vi "Format JSON Object.vi"(7 "Alphabetical Sort":bool, 8 "error in (no error)":errorcluster, 9 "Pretty Print?":bool, 10 "JSON elements":string[](array[string]), 11 "Names":string[](array[string])) -> (0 "error out":errorcluster, 3 "JSON Object Text out":string)   [LabVIEW 2017, in "JSONtext.lvlib"]
uses:
  JSONtext.lvlib
  <vilib>/JDP Science/JDP Science Common Utilities/Trim Whitespace__JDP.vi
  quote and escape json string 2.vi
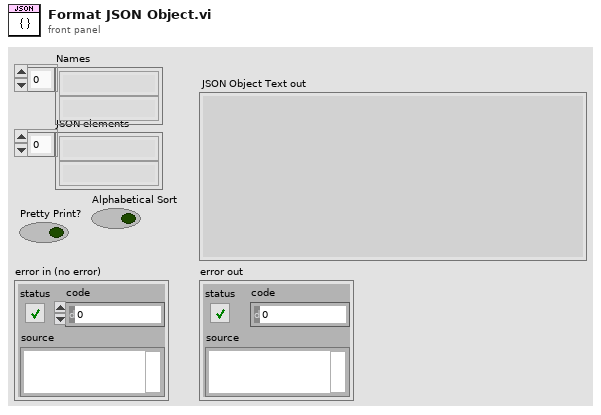
[diagram p1: front panel]
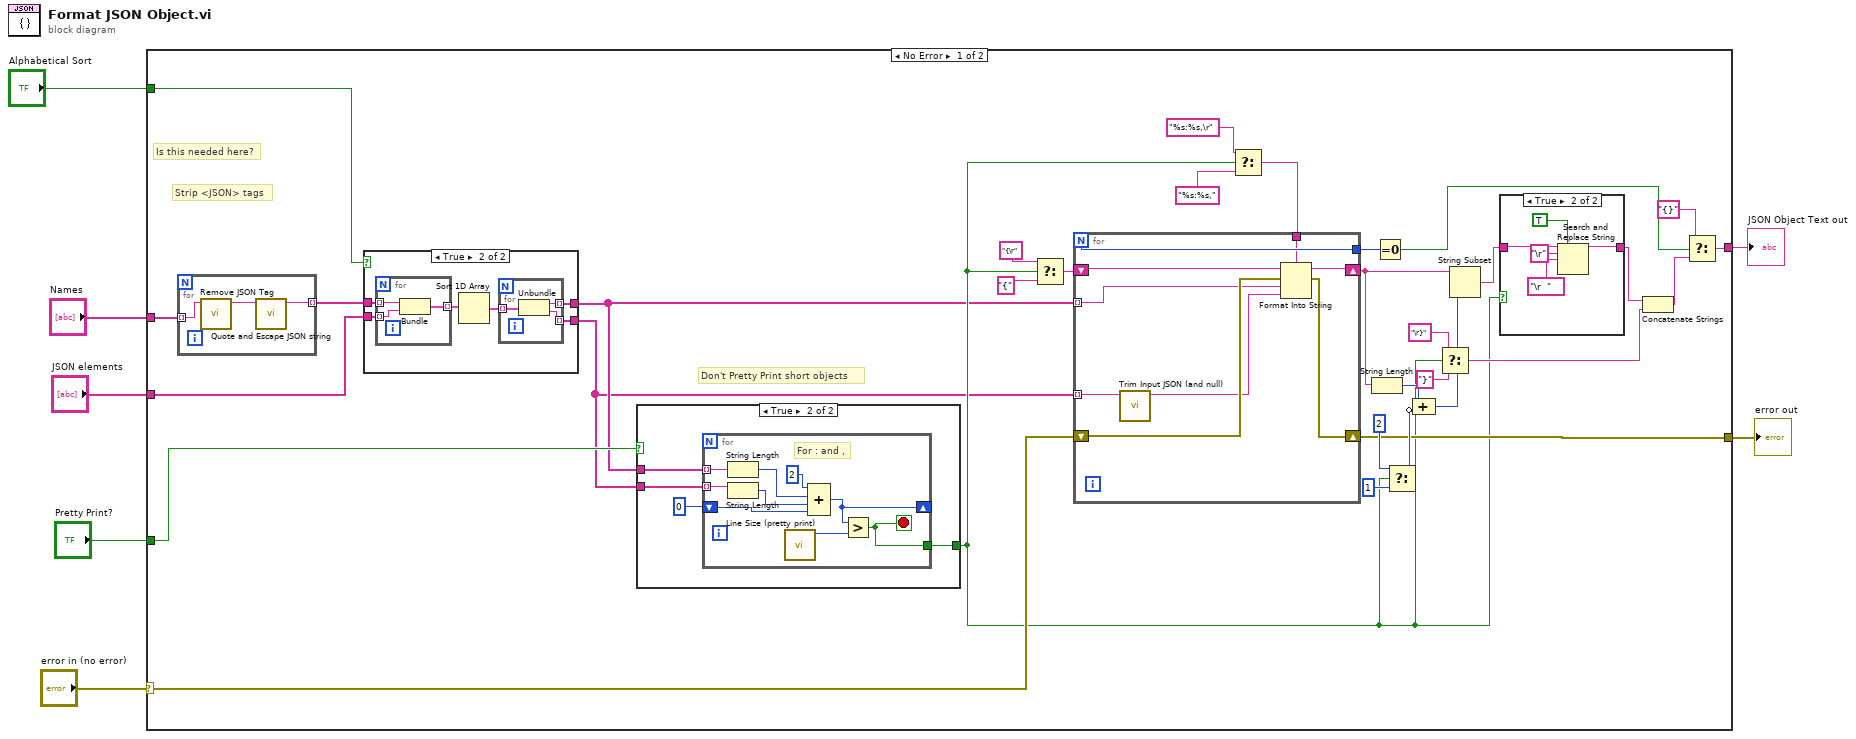
[diagram p0: block diagram]
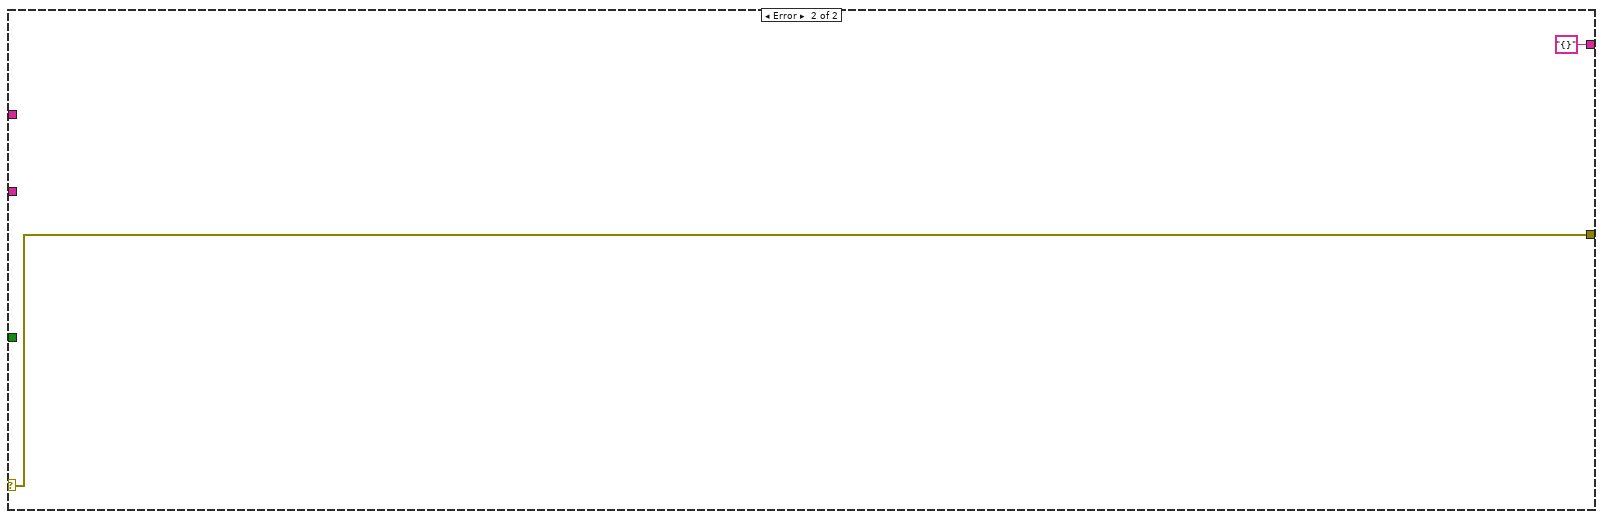
[diagram p5: hidden frame]
diagram:
  n1 = case shown="No Error" "error in (no error)" {
    selector: "error in (no error)" -> [w39 w86]
    tunnel: [w32 "{}" ("t")] -> w6
    tunnel: [w16 w86] -> w5
    tunnel: "Pretty Print?" -> [w15 _]
    tunnel: "Names" -> [w13 _]
    tunnel: "JSON elements" -> [w11 _]
    tunnel: "Alphabetical Sort" -> [w8 _]
    frame No Error {
      # "Is this needed here?"
      # "Don't Pretty Print short objects"
      # "Strip <JSON> tags"
      n2 = for {
        tunnel: w13 -> [w55] mode=indexing
        tunnel: [w54] -> w12 mode=indexing
        n3 = call "Remove JSON Tag.vi"("Name"=w55) -> ("Name (tag stripped)"=w56:string)  [unwired: 9 in, 1 out]
        n4 = call "Quote and Escape JSON string.vi"("Plain Text"=w56) -> ("<JSON>"=w54:string)  [unwired: 10 in]
      }
      n5 = case shown="True" w8 {
        tunnel: w12 -> [w41 w47]
        tunnel: w11 -> [w40 w46]
        tunnel: [w41 w43] -> w10
        tunnel: [w40 w42] -> w9
        frame False {
        }
        frame True {
          n6 = for {
            tunnel: w47 -> [w53] mode=indexing
            tunnel: w46 -> [w52] mode=indexing
            tunnel: [w51] -> w45 mode=indexing
            n7 = Bundle("<JSON>"=w53, "String"=w52) -> (w51:cluster{"<JSON>":string, "String":string})  [unwired: 1 in]
          }
          n8 = Sort 1D Array(array=w45) -> (sorted array=w44:cluster{"<JSON>":string, "String":string}[])
          n9 = for {
            tunnel: w44 -> [w50] mode=indexing
            tunnel: [w49] -> w42 mode=indexing
            tunnel: [w48] -> w43 mode=indexing
            n10 = Unbundle(w50) -> ("<JSON>"=w48:string, "String"=w49:string)
          }
        }
      }
      n11 = case shown="True" w15 {
        tunnel: w9 -> [_ w60]
        tunnel: w10 -> [_ w59]
        tunnel: [_ w57] -> w14
        frame False {
        }
        frame True {
          n12 = for {
            tunnel: w60 -> [w68] mode=indexing
            tunnel: w59 -> [w69] mode=indexing
            shift-right: [w66] -> _
            shift-left: 0 -> [w67]
            tunnel: [w65] -> w57
            stop <- w65 stop-if-true
            # "For : and ,"
            n13 = String Length(string=w69) -> (length=w62:i32)
            n14 = String Length(string=w68) -> (length=w63:i32)
            n15 = call "Line Size (pretty print).vi"() -> ("Line Size"=w64:i32)  [unwired: 11 in]
            n16 = Compound Arithmetic op=ADD(2 ("value"), w62, w63, w67) -> (w66:i32)
            n17 = Greater?(x=w66, y=w64) -> (0:w65:bool)
          }
        }
      }
      n18 = Select(t="{\r", s=w14, f="{") -> (s? t:f=w24:string)
      n19 = Select(t="%s:%s,\r" ("format string"), s=w14, f="%s:%s," ("format string")) -> (s? t:f=w35:string)
      n20 = for {
        N -> [w81]
        tunnel: w10 -> [w78] mode=indexing
        tunnel: w9 -> [w77] mode=indexing
        shift-right: [w82] -> w22
        shift-left: w24 -> [w84]
        shift-right: [w83] -> w16
        shift-left: w39 -> [w79]
        tunnel: [w81] -> w17
        tunnel: w35 -> [w80]
        n21 = call "Trim Input JSON (and null).vi"("JSON Input"=w77) -> ("<JSON>"=w76:string)  [unwired: 10 in]
        n22 = Format Into String(format string=w80, initial string=w84, error in=w79, w78, w76) -> (resulting string=w82:string, error out=w83:errorcluster)
      }
      n23 = String Length(string=w22) -> (length=w21:i32)
      n24 = Equal To 0?(x=w17) -> (x = 0?=w18:bool)
      n25 = Select(t=2, s=w14, f=1) -> (s? t:f=w38:i32)
      n26 = Compound Arithmetic op=ADD(w21, invert w38) -> (w23:i32)
      n27 = Select(t="\r}" ("substring (\"\")"), s=w14, f="}" ("substring (\"\")")) -> (s? t:f=w27:string)
      n28 = String Subset(string=w22, length (rest)=w23) -> (substring=w29:string)  [unwired: 1 in]
      n29 = case shown="True" w14 {
        tunnel: w29 -> [w70 w75]
        tunnel: [w70 w74] -> w30
        frame False {
        }
        frame True {
          n30 = Search and Replace String(replace all?=TRUE ("replace all? (F)"), input string=w75, search string="\r", replace string="\r  " ("search string")) -> (result string=w74:string)  [unwired: 4 in, 3 out]
        }
      }
      n31 = Concatenate Strings(w30, w27) -> (w31:string)
      n32 = Select(t="{}", s=w18, f=w31) -> (s? t:f=w32:string)
    }
    frame Error {
    }
  }
  "JSON Object Text out" <- w6
  "error out" <- w5
